vi "TestFtp.vi"() -> ()   [LabVIEW 2017]
uses:
  <vilib>/Utility/file.llb/Read Delimited Spreadsheet (DBL).vi
  data_txt/hour_txt.vi
  data_txt/year_txt.vi
  data_txt/month_txt.vi
  data_txt/date_txt.vi
  giotxt.vi
  <vilib>/FTP/NI_FTP.lvlib
panel:
  out "first row":dbl[](array[numeric])
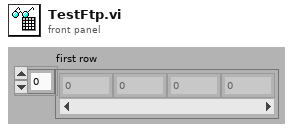
[diagram p1: front panel]
types:
  T1 = typedef "LVDateTimeRec.ctl" = cluster{"fractional second":dbl, "second":i32, "minute":i32, "hour":i32, "day of month":i32, "month":i32, "year":i32, "day of week":i32, "day of year":i32, "DST":i32}
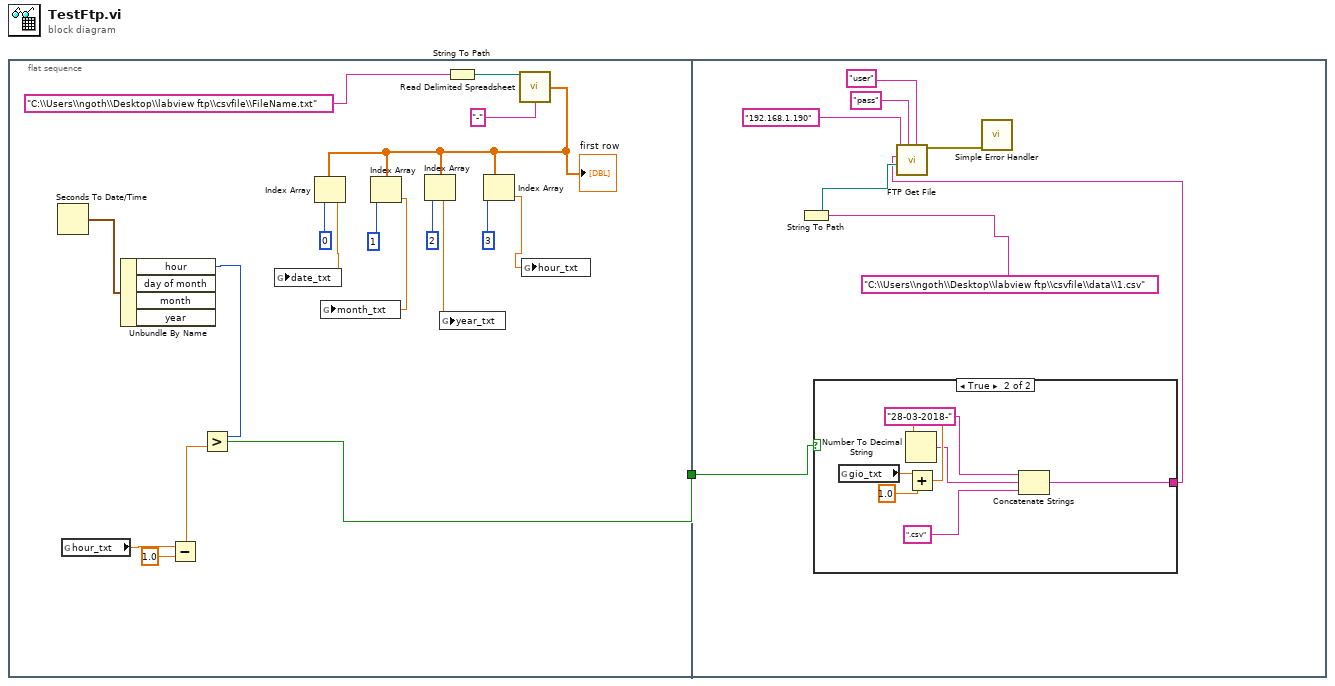
[diagram p0: block diagram]
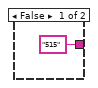
[diagram p2: hidden frame]
diagram:
  n1 = flat-sequence {
    tunnel: [w12] -> w1
    tunnel: w1 -> [w20]
    frame #0 {
      n2 = Seconds To Date/Time() -> (date time rec=w16:T1)  [unwired: 2 in]
      n3 = global read "hour_txt.vi" "hour_txt"() -> (w3:dbl)
      n4 = Unbundle By Name(w16) -> ("hour"=w14:i32)  [unwired: 3 out]
      n5 = Subtract(x=w3, y=1.0) -> (x-y=w13:dbl)
      n6 = Greater?(x=w14, y=w13) -> (0:w12:bool)
      n7 = String To Path(string="C:\\Users\\ngoth\\Desktop\\labview ftp\\csvfile\\FileName.txt") -> (path=w17:path)
      n8 = call-poly <vilib>:"Read Delimited Spreadsheet.vi"("file path (dialog if empty)"=w17, "delimiter (\\t)"="-" ("delimiter (\\t)")) -> ("first row"=w11:dbl[])  [unwired: 8 in, 5 out]
      "first row" <- w11
      n9 = Index Array(array=w11, index=0) -> (element=w6:dbl)
      n10 = global write "date_txt.vi" "date_txt"(w6) -> ()
      n11 = Index Array(array=w11, index=1) -> (element=w5:dbl)
      n12 = global write "month_txt.vi" "month_txt"(w5) -> ()
      n13 = Index Array(array=w11, index=2) -> (element=w7:dbl)
      n14 = global write "year_txt.vi" "year_txt"(w7) -> ()
      n15 = Index Array(array=w11, index=3) -> (element=w4:dbl)
      n16 = global write "hour_txt.vi" "hour_txt"(w4) -> ()
    }
    frame #1 {
      n17 = String To Path(string="C:\\Users\\ngoth\\Desktop\\labview ftp\\csvfile\\data\\1.csv") -> (path=w22:path)
      n18 = case shown="True" w20 {
        tunnel: ["515" w29] -> w21
        frame False {
        }
        frame True {
          n19 = global read "giotxt.vi" "gio_txt"() -> (w33:dbl)
          n20 = Add(x=w33, y=1.0) -> (x+y=w31:dbl)
          n21 = Number To Decimal String(number=w31) -> (decimal integer string=w30:string)  [unwired: 1 in]
          n22 = Concatenate Strings("28-03-2018-" ("string"), w30, ".csv" ("string")) -> (w29:string)
        }
      }
      n23 = call <vilib>:"FTP Get File.vi"("password"="user" ("user"), "user"="pass", "local path"=w22, "remote path"=w21, "host"="192.168.1.190") -> ("error out"=w27:errorcluster)  [unwired: 5 in, 1 out]
      n24 = call <vilib>:"Simple Error Handler.vi"("error in (no error)"=w27) -> ()  [unwired: 4 in, 5 out]
    }
  }
